vi "Change Power Level.vi"(8 "error in (no error)":errorcluster, 10 "Change Power Level Cluster":T2, 11 "Message Handling Cluster in":T1) -> (0 "error out":errorcluster, 3 "Message Handling Cluster out":T1)   [LabVIEW 2024]
uses:
  Controls/Clusters/Change Power Level Cluster.ctl
  Controls/Clusters/Message Handling Cluster.ctl
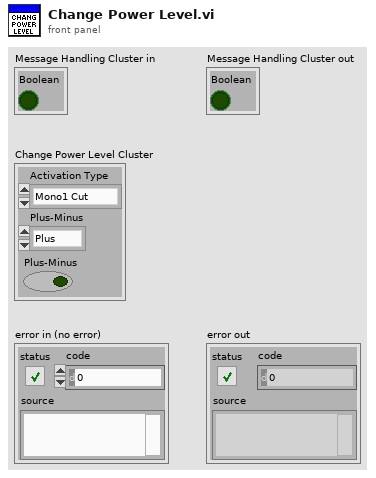
[diagram p1: front panel]
types:
  T1 = typedef "Message Handling Cluster.ctl" = cluster{"Boolean":bool}
  T2 = typedef "Change Power Level Cluster.ctl" = cluster{"Activation Type":enum16{"Mono1 Cut", "Mono1 Coag", "Mono2 Cut", "Mono2 Coag", "Bipolar"}, "Plus-Minus":enum16{"Plus", "Minus"}, "Plus-Minus":bool}
  T3 = enum16{"Mono1 Cut", "Mono1 Coag", "Mono2 Cut", "Mono2 Coag", "Bipolar"}
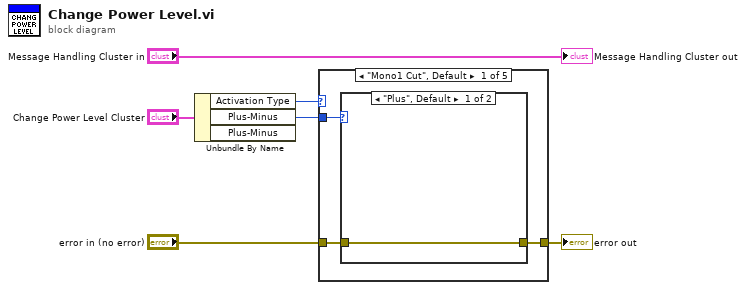
[diagram p0: block diagram]
diagram:
  n1 = Unbundle By Name("Change Power Level Cluster") -> ("Activation Type"=w4:T3, "Plus-Minus"=w3:enum16{"Plus", "Minus"})  [unwired: 1 out]
  n2 = case shown="\"Mono1 Cut\", Default" w4 {
    tunnel: w3 -> [w9 w14 w19 w24 w29]
    tunnel: [w8 w13 w18 w23 w28] -> w2
    tunnel: "error in (no error)" -> [w7 w12 w17 w22 w27]
    frame "Mono1 Cut", Default {
      n3 = case shown="\"Plus\", Default" w9 {
        tunnel: [w10 w11] -> w8
        tunnel: w7 -> [w10 w11]
        frame "Plus", Default {
        }
        frame "Minus" {
        }
      }
    }
    frame "Mono1 Coag" {
      n4 = case shown="\"Plus\", Default" w14 {
        tunnel: [w15 w16] -> w13
        tunnel: w12 -> [w15 w16]
        frame "Plus", Default {
        }
        frame "Minus" {
        }
      }
    }
    frame "Mono2 Cut" {
      n5 = case shown="\"Plus\", Default" w19 {
        tunnel: [w20 w21] -> w18
        tunnel: w17 -> [w20 w21]
        frame "Plus", Default {
        }
        frame "Minus" {
        }
      }
    }
    frame "Mono2 Coag" {
      n6 = case shown="\"Plus\", Default" w24 {
        tunnel: [w25 w26] -> w23
        tunnel: w22 -> [w25 w26]
        frame "Plus", Default {
        }
        frame "Minus" {
        }
      }
    }
    frame "Bipolar" {
      n7 = case shown="\"Plus\", Default" w29 {
        tunnel: [w30 w31] -> w28
        tunnel: w27 -> [w30 w31]
        frame "Plus", Default {
        }
        frame "Minus" {
        }
      }
    }
  }
  "error out" <- w2
  "Message Handling Cluster out" <- "Message Handling Cluster in"
